vi "Set temperature.vi"(8 "error in (no error)":errorcluster, 11 "CCD in":refnum<class "CCD.lvclass">) -> (0 "error out":errorcluster, 3 "CCD out":refnum<class "CCD.lvclass">)   [LabVIEW 2018, in "CCD.lvclass"]
uses:
  CCD.lvclass
  CCD.lvclass/CCD.ctl
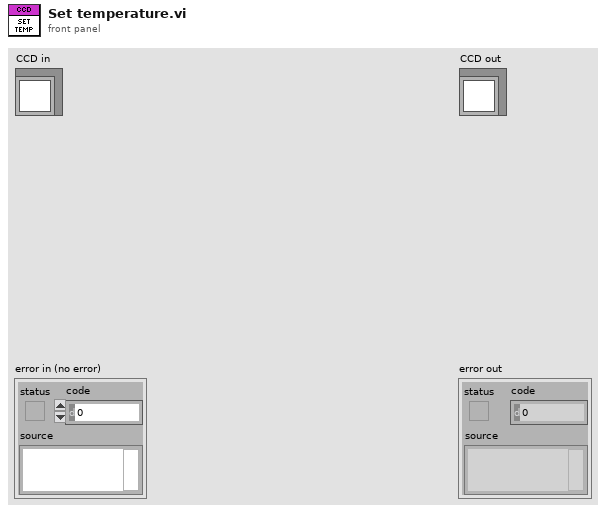
[diagram p1: front panel]
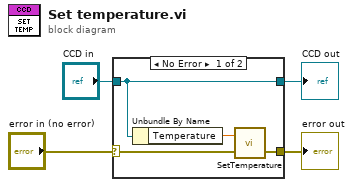
[diagram p0: block diagram]
diagram:
  n1 = case shown="No Error" "error in (no error)" {
    selector: "error in (no error)" -> [w8 w10]
    tunnel: [w7 w10] -> w2
    tunnel: [w6 w9] -> w1
    tunnel: "CCD in" -> [w6 w9]
    frame No Error {
      n2 = Unbundle By Name(w6) -> ("Temperature"=w5:dbl)
      n3 = call <userlib>:"SetTemperature.vi"("error in (no error)"=w8, "temperature"=w5) -> ("error out"=w7:errorcluster)  [unwired: 1 out]
    }
    frame Error {
    }
  }
  "error out" <- w2
  "CCD out" <- w1
